vi "UHR-Fleezers Control (host) - 16.2.2v2.vi"() -> ()   [LabVIEW 2014] (continued)
        n2770 = case shown="False" w4007 {
          tunnel: [w4012 w4019] -> w4009
          tunnel: w4004 -> [w4010 w4019]
          frame False {
            n2771 = local read "Trap Pos FB Monitor\nT1 or T2"() -> (w4015:bool)
            n2772 = local read "Trap X AI1 (DMA)"() -> (w4018:T15)
            n2773 = Unbundle By Name(w4018) -> ("Set 1"=w4017:fxp<+/-,16,1>, "Set 2"=w4016:fxp<+/-,16,1>)
            n2774 = Select(t=w4017, s=w4015, f=w4016) -> (s? t:f=w4014:fxp<+/-,16,1>)
            n2775 = Not(x="Set SP Using...") -> (.not. x?=w4011:bool)
            n2776 = Select(t=w4010, s=w4011, f=w4014) -> (s? t:f=w4012:fxp<+/-,16,1>)
          }
          frame True {
          }
        }
        n2777 = xnode "Read/Write Control"("FPGA VI Reference In"=w4006, "error in"=w4005, "Trap Pos. FB SP"=w4009) -> ()  [unwired: 2 out]
        n2778 = local write "Trap Pos FB SP"(w4009) -> ()
      }
      event "Trap Pos. FB Out Scale 2^n": Value Change {
        n2779 = event-data() -> ()  [unwired: 7 out]
        n2780 = Scale By Power Of 2(n="Trap Pos. FB Out Scale 2^n", x=ext 1.0) -> (x*2^n=w4020:ext)
        n2781 = property on="Trap Pos. FB Mult Factor" class="DigNum (strict)"("Val(Sgnl)"=w4020) -> ()  [unwired: 2 in, 2 out]
      }
      event "Trap Pos FB Int Count": Value Change {
        n2782 = event-data() -> ()  [unwired: 7 out]
        n2783 = xnode "Read/Write Control"("FPGA VI Reference In"=w4023, "Trap Pos FB Int Count"="Trap Pos FB Int Count") -> ()  [unwired: 1 in, 2 out]
      }
      event "Display Saved Data": Value Change {
        n2784 = event-data() -> ()  [unwired: 7 out]
        n2785 = case shown="\"Amp Current\"" "Display Saved Data" {
          frame "Bead Seperation", Default {
            n2786 = property on="Amp current" class="WFGraph (strict)"("Visible"=FALSE) -> ()  [unwired: 2 in, 2 out]
            n2787 = property on="Trap Delta Graph" class="WFGraph (strict)"("Visible"=TRUE) -> ()  [unwired: 2 in, 2 out]
            n2788 = property on="Saved trap pos" class="WFGraph (strict)"("Visible"=FALSE) -> ()  [unwired: 2 in, 2 out]
          }
          frame "Amp Current" {
            n2789 = property on="Saved trap pos" class="WFGraph (strict)"("Visible"=FALSE) -> ()  [unwired: 2 in, 2 out]
            n2790 = property on="Trap Delta Graph" class="WFGraph (strict)"("Visible"=FALSE) -> ()  [unwired: 2 in, 2 out]
            n2791 = property on="Amp current" class="WFGraph (strict)"("Visible"=TRUE) -> ()  [unwired: 2 in, 2 out]
          }
          frame "Trap Position" {
            n2792 = property on="Saved trap pos" class="WFGraph (strict)"("Visible"=TRUE) -> ()  [unwired: 2 in, 2 out]
            n2793 = property on="Trap Delta Graph" class="WFGraph (strict)"("Visible"=FALSE) -> ()  [unwired: 2 in, 2 out]
            n2794 = property on="Amp current" class="WFGraph (strict)"("Visible"=FALSE) -> ()  [unwired: 2 in, 2 out]
          }
        }
      }
      event "Calibration": Value Change {
        n2795 = event-data() -> ()  [unwired: 7 out]
        n2796 = local read "X or Y?"() -> (w4051:bool)
        n2797 = local read "Calibration"() -> (w4048:u16)
        n2798 = Select(t="X" ("Label.Text"), s=w4051, f="Y" ("Label.Text")) -> (s? t:f=w4045:string)
        n2799 = case shown="0, Default" w4048 {
          tunnel: ["Position (V)" ("Label.Text") "Position (nm)" ("Label.Text") "Force (pN)" ("Label.Text")] -> w4042
          tunnel: [" (V)" ("Label.Text") " (nm)" ("Label.Text") " (pN)" ("Label.Text")] -> w4039
          frame 0, Default {
          }
          frame 1 {
          }
          frame 2 {
          }
        }
        n2800 = Concatenate Strings("T1 " ("Label.Text"), w4045) -> (w4041:string)
        n2801 = Concatenate Strings("T2 " ("Label.Text"), w4045) -> (w4040:string)
        n2802 = property on="Force" class="WFChart (strict)"("YScale.NameLbl.Text"=w4042) -> ()  [unwired: 2 in, 2 out]
        n2803 = Concatenate Strings("Mean" ("Label.Text"), w4039) -> (w4038:string)
        n2804 = Concatenate Strings(w4041, w4039) -> (w4037:string)
        n2805 = Concatenate Strings(w4040, w4039) -> (w4036:string)
        n2806 = Concatenate Strings("Difference" ("Label.Text"), w4039) -> (w4035:string)
        n2807 = property on="Mean" class="DigNum (strict)"("Caption.Text"=w4038) -> ()  [unwired: 2 in, 2 out]
        n2808 = property on="T1 X" class="DigNum (strict)"("Caption.Text"=w4037) -> ()  [unwired: 2 in, 2 out]
        n2809 = property on="T2 X" class="DigNum (strict)"("Caption.Text"=w4036) -> ()  [unwired: 2 in, 2 out]
        n2810 = property on="Difference" class="DigNum (strict)"("Caption.Text"=w4035) -> ()  [unwired: 2 in, 2 out]
      }
      event "Base N trap periods", "Period scale factor", "Trap osc amp (MHz)", "Cal sets to save", "# Samples/trap", "Total Counts (ticks)": Value Change {
        w4063 = u32 0 ("y")
        # "scales 0 to 2pi"
        # "Create vector of trap offset (oscillation) values."
        # "Compute oscillation period as a multiple of the trap period. Should also fit nicely as a factor of the DMA period.\nCompare ticks for accurate commensurability check."
        # "Oscillation frequency needs to be commensurate\nwith the data save time."
        # "Be commensurate with total save time/100 (or so). That way you are guaranteed you can average spectra at least 100x."
        n2811 = event-data() -> ()  [unwired: 7 out]
        n2812 = local read "Total Counts (ticks)"() -> (w4082:u16)
        n2813 = To Unsigned Long Integer(number=w4082) -> (unsigned 32bit integer=w4092:u32)
        n2814 = Multiply "Base osc period (ticks)"(x=w4092, y="Base N trap periods") -> (x*y=w4083:u32)
        n2815 = local read "# Samples/trap"() -> (w4087:u32)
        n2816 = Multiply "Scaled osc period (ticks)"(x=w4083, y="Period scale factor") -> (x*y=w4084:dbl)
        n2817 = Multiply(x="Base N trap periods", y="Period scale factor") -> (x*y=w4075:dbl)
        n2818 = local read "Cal sets to save"() -> (w4088:u32)
        n2819 = To Unsigned Quad Integer(1:w4084) -> (0:w4072:u64)
        n2820 = for "vector 0 to N -1" {
          N: w4075 -> [_]
          tunnel: [w4110] -> w4080 mode=indexing
          i -> [w4110]
        }
        n2821 = Multiply "Ticks/DMA"(x=w4087, y=w4092) -> (x*y=w4091:u32)
        n2822 = Multiply "Scaled osc period (s)"(x=w4072, y=2.5e-08) -> (x*y=w4086:dbl)
        "Trap OSC Period (s)" <- w4086
        n2823 = Reciprocal(x=w4086) -> (1/x=→"A cal freq (Hz)":dbl)
        n2824 = Multiply(x=w4080, y=6.283185307179586) -> (x*y=w4095:dbl[])
        n2825 = Quotient & Remainder(x=w4091, y=w4072) -> (x-y*floor(x/y)=w4064:u64, floor(x/y)=→"N osc / DMA":u64)
        "DMA remainder" <- w4064
        n2826 = Multiply "Total trap ticks"(x=w4088, y=w4091) -> (x*y=w4073:u32)
        n2827 = Divide(x=w4095, y=w4075) -> (x/y=w4096:dbl[])
        n2828 = Sine(x=w4096) -> (sin(x)=w4097:dbl[])
        n2829 = Quotient & Remainder(x=w4073, y=100) -> (x-y*floor(x/y)=w4067:u32, floor(x/y)=w4090:u32)
        "Total save/100 remainder" <- w4067
        n2830 = Multiply "Single period osc vector"(x=w4097, y="Trap osc amp (MHz)") -> (x*y=w4070:dbl[])
        n2831 = Quotient & Remainder(x=w4090, y=w4072) -> (x-y*floor(x/y)=w4066:u64, floor(x/y)=→"N osc/ (total save/100)":u64)
        "(total save/100) /osc period remainder" <- w4066
        n2832 = Quotient & Remainder(x=w4073, y=w4072) -> (x-y*floor(x/y)=w4065:u64, floor(x/y)=w4071:u64)
        "N trap osc periods per save" <- w4071
        "N trap osc periods per save remainder" <- w4065
        n2833 = call "IR AOM freq to word - vec.vi"("Frequency In (double vec, MHz)"=w4070) -> ("Frequency Word Out"=w4069:dbl[])
        n2834 = xnode "Read/Write Control"("FPGA VI Reference In"=w4079, "Trap osc period (pts)"=w4075, "N trap osc periods"=w4071) -> ("FPGA VI Reference Out"=w4078:T25)  [unwired: 1 in, 1 out]
        n2835 = To Quad Integer(1:w4069) -> (0:w4068:i64[])
        n2836 = Equal?(x=w4066, y=w4063) -> (x = y?=w4061:bool)
        n2837 = Equal?(x=w4067, y=w4063) -> (x = y?=w4062:bool)
        n2838 = Equal?(x=w4064, y=w4063) -> (x = y?=w4059:bool)
        n2839 = Equal?(x=w4065, y=w4063) -> (x = y?=w4060:bool)
        n2840 = flat-sequence {
          tunnel: w4068 -> [w4101]
          tunnel: w4078 -> [w4100]
          frame #0 {
            n2841 = for "Write data to fpga memory" {
              tunnel: w4100 -> [w4106]
              tunnel: w4101 -> [w4104] mode=indexing
              i -> [w4105]
              n2842 = xnode "Read/Write Control"("FPGA VI Reference In"=w4106, "Address 2"=w4105, "Data"=w4104, "Ready Write"=TRUE) -> ("FPGA VI Reference Out"=w4102:T25)  [unwired: 1 in, 1 out]
              n2843 = while {
                tunnel: w4102 -> [w4108]
                stop <- w4107 continue-if-true
                n2844 = xnode "Read/Write Control"("FPGA VI Reference In"=w4108) -> ("Ready Write"=w4107:bool)  [unwired: 1 in, 2 out]
              }
            }
            "Writing waveform to fpga memory" <- TRUE ("Writing waveform to fpga memory")
          }
          frame #1 {
            n2845 = local write "Writing waveform to fpga memory"(FALSE ("Writing waveform to fpga memory")) -> ()
          }
        }
        n2846 = Compound Arithmetic op=AND(w4062, w4061, w4060, w4059) -> (→"Good freq?":bool)
      }
      event "Osc trap cont.", "Osc traps", "T1 Osc Enable", "T2 Osc Enable": Value Change {
        n2847 = event-data() -> ()  [unwired: 7 out]
        n2848 = xnode "Read/Write Control"("FPGA VI Reference In"=w4115, "Osc trap cont."="Osc trap cont.", "Osc traps"="Osc traps", "Trap 1 osc enable"="T1 Osc Enable", "Trap 2 osc enable"="T2 Osc Enable") -> ()  [unwired: 1 in, 2 out]
      }
      event "Pressure Pump Voltage (+/-10V)": Value Change {
        n2849 = event-data() -> ()  [unwired: 7 out]
        n2850 = disable-structure shown="Disabled" {
          disable-tunnel: w4116 -> [w4117 _]
          frame Disabled {
            n2851 = disable-structure shown="Enabled" {
              disable-tunnel: w4117 -> [w4120 _]
              frame Enabled {
                n2852 = Divide(x="Pressure Pump Voltage (+/-10V)", y=10.0) -> (x/y=w4118:dbl)
                n2853 = Multiply(x=w4118, y=32767.0) -> ()  [unwired: 1 out]
                n2854 = xnode "Read/Write Control"("FPGA VI Reference In"=w4120) -> ()  [unwired: 2 in, 2 out]
              }
              frame Disabled {
              }
            }
          }
          frame Enabled {
          }
        }
      }
    }
    "error out 2" <- w2711
    n2855 = node-c288() -> ()  [unwired: 2 out]
  }
  n2856 = disable-structure shown="Disabled" {
    frame Disabled {
      n2857 = while "Duncan's play event loop" {
        stop <- w4125 stop-if-true
        n2858 = Create User Event(user event datatype=TRUE ("Boolean")) -> (user event=w4126:refnum<user-event>)  [unwired: 1 in, 1 out]
        n2859 = Create User Event(user event datatype=TRUE ("Boolean")) -> (user event=w4132:refnum<user-event>)  [unwired: 1 in, 1 out]
        n2860 = global write "Global for fluorescence simulation mean (30 samples), (power series).vi" "Red Signal"(w4126) -> ()
        n2861 = global write "Global for fluorescence simulation mean (30 samples), (power series).vi" "Green Signal"(w4132) -> ()
        n2862 = register-events(w4132, w4126) -> (reference out=w4131:refnum<event-registration>)  [unwired: 2 in, 1 out]
        n2863 = event shown="[1] \"Start assembly line\": Value Change" {
          selector: w4131 -> [_ _ _ _]
          dyn-events: _ -> [_ _ _ _]
          timeout: 100 -> [_ _ _ _]
          event Timeout {
            n2864 = event-data() -> ()  [unwired: 1 in, 2 out]
          }
          event "Start assembly line": Value Change {
            n2865 = event-data() -> ("OldVal"=w4134:bool)  [unwired: 1 in, 4 out]
            n2866 = case shown="True" w4134 {
              selector: w4134 -> [_ w4135]
              frame False {
              }
              frame True {
                n2867 = property on="Move to Position 3" class="Bool"("Val(Sgnl)"=w4135) -> ()  [unwired: 2 in, 2 out]
                n2868 = case shown="1" "Numeric" {
                  frame 0, Default {
                  }
                  frame 1 {
                    n2869 = property on="Green Laser ON" class="Bool (strict)"("Val(Sgnl)"=TRUE ("Value (Signaling)")) -> ()  [unwired: 2 in, 2 out]
                  }
                  frame 2 {
                    n2870 = property on="Red Laser ON" class="Bool (strict)"("Val(Sgnl)"=TRUE) -> ()  [unwired: 2 in, 2 out]
                  }
                }
              }
            }
          }
          event User Event {
            n2871 = event-data() -> ("Boolean"=w4139:bool)  [unwired: 1 in, 3 out]
            "Green Fluorophore" <- w4139
            n2872 = property on="Start assembly line" class="Bool"("Val(Sgnl)"=w4139) -> ()  [unwired: 2 in, 2 out]
          }
          event User Event {
            n2873 = event-data() -> ("Boolean"=w4140:bool)  [unwired: 1 in, 3 out]
            "Red Fluorophore" <- w4140
            n2874 = property on="Start assembly line" class="Bool"("Val(Sgnl)"=w4140) -> ()  [unwired: 2 in, 2 out]
          }
        }
        n2875 = property on="Get Fluorophore" class="Bool (strict)"("Val(Sgnl)"="Get Fluorophore") -> ()  [unwired: 2 in, 2 out]
        n2876 = Wait (ms)(milliseconds to wait=u32 100) -> ()  [unwired: 1 out]
        n2877 = local read "Stop All"() -> (w4124:bool)
        n2878 = Or(x=w4124, y="stop") -> (x .or. y?=w4125:bool)
      }
    }
    frame Enabled {
    }
  }
  n2879 = flat-sequence "Video" {
    tunnel: [w4151] -> w75
    tunnel: w75 -> [w4192]
    frame #0 {
      w4141 = FALSE ("File open?")
      n2880 = while {
        stop <- w4143 continue-if-true
        n2881 = call "Close Video Capture.vi"() -> ("error code OUT"=w4145:i32)
        n2882 = Equal?(x=w4145, y=0) -> (x = y?=w4143:bool)
      }
      n2883 = local write "New Video File"(w4141) -> ()
      n2884 = local write "File open?"(w4141) -> ()
      n2885 = local write "Save Video"(w4141) -> ()
      n2886 = local write "Stop All"(FALSE ("Stop All")) -> ()
    }
    frame #1 {
      n2887 = call "DMR_Init.vi"() -> ()  [unwired: 3 out]
    }
    frame #2 {
      w4146 = "DE245428202"  # MSU fleezers card #
      (unwired) "DE019116701"  # Illinois fleezers card #
      # "Setting the destination format to Mono8 makes sure that the image can be displayed in the intensity plot."
      n2888 = call "DMR_GetDevice.vi"("search string IN"=w4146) -> ("device handle OUT"=w4169:i32)  [unwired: 4 in, 2 out]
      n2889 = call "DMR_OpenDevice.vi"("device handle IN"=w4169) -> ("driver handle OUT"=w4152:i32)  [unwired: 4 out]
      n2890 = call "DMR_FindList.vi"("flags IN"=u32 0 ("flags"), "list name IN"="" ("String"), "list type IN"=T41."camera descriptions", "driver handle IN"=w4152) -> ("list handle OUT"=w4155:i32)  [unwired: 2 out]
      n2891 = call "DMR_FindList.vi"("flags IN"=u32 0 ("flags"), "list name IN"="Base", "list type IN"=T41."setting", "driver handle IN"=w4152) -> ("list handle OUT"=w4153:i32)  [unwired: 2 out]
      n2892 = call "OBJ_GetHandle.vi"("object name IN"="VideoStandard", "list handle IN"=w4155) -> ("object handle OUT"=w4149:i32)  [unwired: 3 out]
      n2893 = call "OBJ_GetHandle.vi"("object name IN"="PixelFormat", "list handle IN"=w4153) -> ("object handle OUT"=w4163:i32)  [unwired: 3 out]
      n2894 = call "OBJ_SetS.vi"("value index IN"=0, "value IN"="NTSC M", "object handle IN"=w4149) -> ()  [unwired: 2 out]
      n2895 = call "OBJ_SetS.vi"("value index IN"=0, "value IN"="Mono8" ("value"), "object handle IN"=w4163) -> ()  [unwired: 2 out]
      n2896 = call "OBJ_GetHandle.vi"("object name IN"="VideoChannel", "list handle IN"=w4153) -> ("object handle OUT"=w4159:i32)  [unwired: 3 out]
      n2897 = while {
        tunnel: [w4173] -> w4151
        tunnel: w4152 -> [w4170]
        stop <- w4171 continue-if-true
        n2898 = call "DMR_ImageRequestSingle.vi"("request control IN"=0, "driver handle IN"=w4170) -> ("error code OUT"=w4172:i32, "driver handle OUT"=w4173:i32)  [unwired: 2 out]
        n2899 = Equal To 0?(x=w4172) -> (x = 0?=w4171:bool)
      }
      n2900 = call "OBJ_SetI.vi"("value index IN"=0, "value IN"="Video channel", "object handle IN"=w4159) -> ()  [unwired: 2 out]
    }
    frame #3 {
      w4180 = T22 0 items=["Grayscale (U8)", "Grayscale (I16)", "Grayscale (SGL)", "Complex (CSG)", "RGB (U32)", "HSL (U32)", "RGB (U64)"] ("Image Type")
      w4188 = T22 0 items=["Grayscale (U8)", "Grayscale (I16)", "Grayscale (SGL)", "Complex (CSG)", "RGB (U32)", "HSL (U32)", "RGB (U64)"] ("Image Type")
      n2901 = call "IMAQ AVI2 Get Codec Names"() -> ("Codec Names"=w4175:string[])  [unwired: 10 in, 1 out]
      "Installed Codec Names" <- w4175
      n2902 = for "Create Greyscale map" {
        N: 256 -> [_]
        tunnel: [w4194] -> w4177 mode=indexing
        workers-P: _ -> [_]
        i -> [w4197]
        n2903 = To Unsigned Byte Integer(number=w4197) -> (unsigned 8bit integer=w4193:u8)
        n2904 = Join Numbers(hi=w4193, lo=w4193) -> ((hi.lo)=w4196:u16)
        n2905 = Join Numbers(hi=w4193, lo=w4193) -> ((hi.lo)=w4195:u16)
        n2906 = Join Numbers(hi=w4196, lo=w4195) -> ((hi.lo)=w4194:u32)
      }
      n2907 = property on="Codec choice" class="CmbBox"("Strings[]"=w4175) -> ()  [unwired: 2 in, 2 out]
      n2908 = call "IMAQ Create"("Image Name"="Scaled video", "Image Type"=w4180) -> ("New Image"=w4179:T2)  [unwired: 2 in, 2 out]
      n2909 = call "IMAQ Create"("Image Name"="Main video", "Image Type"=w4188) -> ("New Image"=w4189:T2)  [unwired: 2 in, 2 out]
      n2910 = node-c288(0 ("Processor")) -> (w4187:T28)  [unwired: 3 out]
      n2911 = Initialize Array(u32 0 ("Window Number (0...15)"), 480 ("dimension size"), 640 ("dimension size")) -> (w4182:u32[][])
      n2912 = timed-loop {
        tunnel: w4192 -> [w4214]
        tunnel: [w4213] -> w4191
        tunnel: w4189 -> [w4212]
        timing: w4187 -> [_]
        timing-out: [_] -> w4186
        tunnel: w4182 -> [w4205]
        tunnel: w4179 -> [w4203]
        tunnel: w4177 -> [w4202]
        stop <- w4204 stop-if-true
        # "This block performs the \nactual image capture."
        n2913 = node-c288() -> (→"Finished Late? [i-1]":bool)  [unwired: 5 out]
        n2914 = local read "Stop All"() -> (w4204:bool)
        n2915 = feedback #2(T42 refnum ("AVI Refnum")) -> (w4210:T42)
        n2916 = case shown="True" "New Video File" {
          tunnel: [w4227 w4228] -> w4201
          tunnel: w4210 -> [w4227 w4229]
          frame False {
          }
          frame True {
            n2917 = flat-sequence {
              tunnel: w4229 -> [w4231]
              tunnel: [w4233] -> w4228
              frame #0 {
                n2918 = local read "File open?"() -> (w4230:bool)
                n2919 = case shown="True" w4230 {
                  tunnel: w4231 -> [_ w4232]
                  frame False {
                  }
                  frame True {
                    n2920 = call "IMAQ AVI2 Close"("AVI Refnum"=w4232) -> ()  [unwired: 10 in, 1 out]
                  }
                }
              }
              frame #1 {
                n2921 = local write "New Video File"(FALSE ("New Video File")) -> ()
                n2922 = call "Create new save file.vi"("Ext"=".avi" ("string"), "Index In"="Video Index") -> ("Path Out"=w4236:path, "Index Out"=w4238:dbl)  [unwired: 1 in]
                "Path Out" <- w4236
                n2923 = local write "Video Index"(w4238) -> ()
                n2924 = call "IMAQ AVI2 Create"("Codec"="Codec choice", "Frames Per Second"=u32 30, "AVI Path"=w4236) -> ("AVI Refnum"=w4233:T42)  [unwired: 7 in, 1 out]
                "File open?" <- TRUE ("Files open?")
              }
            }
          }
        }
        n2925 = feedback-in #2(w4201) -> ()
        n2926 = call "DMR_ImageRequestWaitFor.vi"("queue number IN"=0, "timeout(ms) IN"=500, "driver handle IN"=w4214) -> ("error code OUT"=w4218:i32, "request number OUT"=w4215:i32, "driver handle OUT"=w4216:i32)
        n2927 = Equal To 0?(x=w4218) -> (x = 0?=w4217:bool)
        n2928 = Reciprocal(x="Video Capture Rate (Hz)") -> (1/x=w4208:dbl)
        n2929 = Multiply(x=w4208, y=1000.0) -> (x*y=w4206:dbl)
        n2930 = case shown="True" w4217 {
          tunnel: w4216 -> [w4242 w4279]
          tunnel: w4215 -> [_ w4278]
          tunnel: [w4242 w4275] -> w4213
          tunnel: w4212 -> [_ w4261]
          tunnel: w4205 -> [_ w4264]
          tunnel: w4201 -> [_ w4244]
          tunnel: w4203 -> [_ w4258]
          tunnel: w4202 -> [_ w4257]
          frame False {
          }
          frame True {
            w4269 = u32 0 ("X-offset IN")
            n2931 = call "DMR_GetImageRequestBufferData.vi"("driver handle IN"=w4279, "request number IN"=w4278) -> ("width OUT"=w4268:i32, "height OUT"=w4267:i32, "driver handle OUT"=w4274:i32, "request number OUT"=w4273:i32, "bytes per pixel OUT"=w4270:i32)  [unwired: 13 out]
            n2932 = call "DMR_GetImageRequestBufferImageData.vi"("driver handle IN"=w4274, "request number IN"=w4273, "bytes per pixel IN"=w4270, "X-offset IN"=w4269, "Y-offset IN"=w4269, "height IN"=w4267, "width IN"=w4268) -> ("driver handle OUT"=w4272:u32, "request number OUT"=w4271:u32, "image OUT"=w4250:u32[][])  [unwired: 10 out]
            n2933 = Transpose 2D Array(2D array=w4250) -> (transposed array=w4256:u32[][])
            n2934 = Select(t=w4256, s="Flip Y (or X)", f=w4250) -> (s? t:f=w4255:u32[][])
            n2935 = call "DMR_ImageRequestUnlock.vi"("request number IN"=w4271, "driver handle IN"=w4272) -> ("driver handle OUT"=w4277:i32)  [unwired: 1 in, 2 out]
            n2936 = for {
              tunnel: w4255 -> [w4314] mode=indexing
              tunnel: [w4313] -> w4253 mode=indexing
              n2937 = Reverse 1D Array(array=w4314) -> (reversed array=w4313:u32[])
            }
            n2938 = call "DMR_ImageRequestSingle.vi"("request control IN"=0, "driver handle IN"=w4277) -> ("driver handle OUT"=w4275:i32)  [unwired: 3 out]
            n2939 = Transpose 2D Array(2D array=w4253) -> (transposed array=w4254:u32[][])
            n2940 = Select(t=w4254, s="Flip Y (or X)", f=w4253) -> (s? t:f=w4251:u32[][])
            n2941 = Select(t=w4251, s="Flip Image", f=w4250) -> (s? t:f=w4248:u32[][])
            n2942 = case shown="True" "Averaging" {
              tunnel: w4248 -> [w4325 w4330]
              tunnel: [w4325 w4329] -> w4262
              tunnel: w4264 -> [_ w4327]
              frame False {
              }
              frame True {
                (unwired) 1
                w4335 = 1
                n2943 = feedback #3(w4327) -> (w4326:u32[][])
                n2944 = Add(x=w4330, y=w4326) -> (x+y=w4331:u32[][])
                n2945 = Select(t=w4327, s="Reset Averaging", f=w4331) -> (s? t:f=w4333:u32[][])
                n2946 = feedback-in #3(w4333) -> ()
                n2947 = feedback #4(w4335) -> (w4328:i32)
                n2948 = Divide(x=w4331, y=w4328) -> (x/y=w4332:dbl[][])
                n2949 = Increment(x=w4328) -> (x+1=w4336:i32)
                n2950 = To Unsigned Long Integer(number=w4332) -> (unsigned 32bit integer=w4329:u32[][])
                n2951 = Select(t=w4335, s="Reset Averaging", f=w4336) -> (s? t:f=w4334:i32)
                n2952 = feedback-in #4(w4334) -> ()
              }
            }
            n2953 = case shown="True" "Zoom video window" {
              tunnel: w4262 -> [_ w4293]
              tunnel: w4258 -> [_ w4292]
              frame False {
              }
              frame True {
                n2954 = To Double Precision Float(number=w4293) -> (double precision float=w4290:dbl[][])
                n2955 = In Range and Coerce(upper limit="Intensity Upper", x=w4290, lower limit="Intensity Lower") -> (coerced(x)=w4289:dbl[][])  [unwired: 1 out]
                n2956 = Subtract(x="Intensity Upper", y="Intensity Lower") -> (x-y=w4286:dbl)
                n2957 = Subtract(x=w4289, y="Intensity Lower") -> (x-y=w4287:dbl[][])
                n2958 = Divide(x=w4287, y=w4286) -> (x/y=w4288:dbl[][])
                n2959 = Multiply(x=255.0, y=w4288) -> (x*y=w4284:dbl[][])
                n2960 = To Unsigned Byte Integer(number=w4284) -> (unsigned 8bit integer=w4291:u8[][])
                n2961 = call "IMAQ ArrayToImage"("Image Pixels (U8)"=w4291, "Image"=w4292) -> ("Image Out"=w4280:T2)  [unwired: 4 in, 5 out]
                n2962 = First Call?() -> (First Call?: T/F=w4281:bool)
                n2963 = case shown="True" w4281 {
                  tunnel: w4280 -> [w4294 w4305]
                  frame False {
                    n2964 = flat-sequence {
                      tunnel: w4294 -> [w4300]
                      frame #0 {
                        w4297 = FALSE ("Get/Set Status? (Set)")
                        w4296 = 0 ("Window Number (0...15)")
                        n2965 = call "IMAQ WindSize"("Get/Set Status? (Set)"=w4297, "Window Number"=w4296) -> ("Width & Height out"=→"Window Size":cluster{"Width":i32, "Height":i32})  [unwired: 4 in, 2 out]
                        n2966 = call "IMAQ WindMove"("Window Number (0...15)"=w4296, "Get/Set Status? (Set)"=w4297) -> ("Coordinates (screen)"=→"Window Position":cluster{"X Position":i32, "Y Position":i32})  [unwired: 3 in, 1 out]
                        n2967 = call "IMAQ WindDraw"("Resize to Image Size? (Y)"=FALSE, "Window Number (0...15)"=w4296, "Image"=w4300) -> ()  [unwired: 7 in, 2 out]
                      }
                      frame #1 {
                        n2968 = call "IMAQ WindZoom 2"("Center Point"="Center Point", "Zoom to Fit? (False)"=FALSE, "Zoom Factor"="Zoom Factor") -> ()  [unwired: 5 in, 4 out]
                      }
                    }
                  }
                  frame True {
                    n2969 = flat-sequence {
                      tunnel: w4305 -> [w4308]
                      tunnel: [w4306] -> w4304
                      tunnel: w4304 -> [w4310]
                      frame #0 {
                        w4307 = TRUE ("Resize to Image Size? (Y)")
                        w4306 = 0 ("Window Number (0...15)")
                        n2970 = call "IMAQ WindNonTearing"("Window Number"=w4306, "NonTearing? (True)"=w4307) -> ()  [unwired: 8 in, 2 out]
                        n2971 = call "IMAQ WindDraw"("Resize to Image Size? (Y)"=w4307, "Window Number (0...15)"=w4306, "Image"=w4308) -> ()  [unwired: 7 in, 2 out]
                      }
                      frame #1 {
                        n2972 = call "IMAQ WindSize"("Scrollbars? (N)"=FALSE, "Width & Height"="Initial Window Size", "Window Number"=w4310) -> ()  [unwired: 3 in, 3 out]
                        n2973 = call "IMAQ WindMove"("Window Number (0...15)"=w4310, "Coordinates (screen)"="Initial Window Position") -> ()  [unwired: 3 in, 2 out]
                      }
                    }
                  }
                }
              }
            }
            n2974 = To Unsigned Byte Integer(number=w4262) -> (unsigned 8bit integer=w4260:u8[][])
            n2975 = call "IMAQ ArrayToImage"("Image Pixels (U8)"=w4260, "Image"=w4261) -> ("Image Out"=w4259:T2)  [unwired: 4 in, 5 out]
            "Primary Video Display" <- w4259
            n2976 = Not(x="Close Video File") -> (.not. x?=w4246:bool)
            n2977 = And(x="Save Video", y=w4246) -> (x .and. y?=w4243:bool)
            n2978 = case shown="True" "Save Image" {
              tunnel: w4260 -> [_ w4339]
              tunnel: w4257 -> [_ w4338]
              frame False {
              }
              frame True {
                n2979 = call <vilib>:"Flatten Pixmap.vi"("colors"=w4338, "8-bit pixmap"=w4339) -> ("image data"=w4345:T43)  [unwired: 4 in, 5 out]
                n2980 = call "Create new save file.vi"("Insert"="video_frame_" ("string"), "Ext"=".bmp" ("string"), "Index In"="Image Index") -> ("Path Out"=w4341:path, "Index Out"=w4346:dbl)
                n2981 = Increment(x=w4346) -> (x+1=w4340:dbl)
                n2982 = local write "Image Index"(w4340) -> ()
                n2983 = call <vilib>:"Write BMP File.vi"("image data"=w4345, "path to BMP file"=w4341) -> ()  [unwired: 1 in, 9 out]
              }
            }
            n2984 = case shown="True" w4243 {
              tunnel: w4244 -> [w4316 w4321]
              tunnel: w4259 -> [_ w4320]
              tunnel: "Close Video File" -> [w4315 _]
              frame False {
                n2985 = case shown="True" w4315 {
                  tunnel: w4316 -> [_ w4317]
                  frame False {
                  }
                  frame True {
                    w4318 = FALSE ("Save Video")
                    n2986 = call "IMAQ AVI2 Close"("AVI Refnum"=w4317) -> ()  [unwired: 10 in, 1 out]
                    n2987 = local write "File open?"(w4318) -> ()
                    n2988 = local write "Save Video"(w4318) -> ()
                  }
                }
              }
              frame True {
                n2989 = local read "File open?"() -> (w4319:bool)
                n2990 = case shown="True" w4319 {
                  tunnel: w4321 -> [_ w4324]
                  tunnel: w4320 -> [_ w4323]
                  frame False {
                    n2991 = local write "New Video File"(TRUE ("New Video File")) -> ()
                  }
                  frame True {
                    n2992 = call "IMAQ AVI2 Write Frame"("Image"=w4323, "AVI Refnum"=w4324) -> ()  [unwired: 7 in, 3 out]
                  }
                }
              }
            }
          }
        }
        n2993 = node-c288(w4206, "Deadline (ms)") -> ()  [unwired: 1 out]
      }
      n2994 = node-c288(w4186) -> ()  [unwired: 1 out]
      n2995 = call "DMR_CloseDevice.vi"("driver handle IN"=w4191) -> ()  [unwired: 1 in, 4 out]
    }
    frame #4 {
      n2996 = call "DMR_Close.vi"() -> ()  [unwired: 1 out]
    }
  }
  n2997 = node-c288(w45) -> ()  [unwired: 1 out]
  n2998 = node-c288(w84) -> ()  [unwired: 1 out]
  n2999 = node-c288(w86) -> ()  [unwired: 1 out]
  n3000 = node-c288(w73) -> ()  [unwired: 1 out]
  n3001 = disable-structure shown="Disabled" {
    disable-tunnel: w77 -> [w4352 _]
    disable-tunnel: w76 -> [w4351 _]
    frame Disabled {
      n3002 = VISA Close(VISA resource name=w4352, error in (no error)=w4351) -> (error out=w4353:errorcluster)
      n3003 = call <vilib>:"Simple Error Handler.vi"("error in (no error)"=w4353) -> ()  [unwired: 1 in, 8 out]
    }
    frame Enabled {
    }
  }
  n3004 = property on="Saved trap pos" class="WFGraph (strict)"("Visible"=FALSE) -> ()  [unwired: 2 in, 2 out]
  n3005 = property on="Trap Delta Graph" class="WFGraph (strict)"("Visible"=TRUE) -> ()  [unwired: 2 in, 2 out]
  n3006 = node-c288(w82) -> ()  [unwired: 1 out]
  n3007 = Unbundle By Name("sound format") -> ("sample rate (S/s)"=w23:dbl)
  n3008 = call <vilib>:"Sound Output Configure.vi"("number of samples/ch"="number of samples/ch", "sample mode"="sample mode", "sound format"="sound format", "device ID"="device ID") -> ("task ID"=w27:T44)  [unwired: 6 in, 1 out]
  n3009 = local read "DMA Update Period (s)"() -> (w24:dbl)
  n3010 = Multiply(x=w24, y=w23) -> (x*y=w22:dbl)
  n3011 = for "Sound time base" {
    N: w22 -> [_]
    tunnel: [w4354] -> w25 mode=indexing
    i -> [w4354]
  }
  n3012 = Reciprocal(x=w23) -> (1/x=w21:dbl)
  n3013 = Multiply(x=w25, y=w21) -> (x*y=w20:dbl[])
  n3014 = timed-loop "Main data acquisition loop (get data, process data for display, and save data to disk)" {
    tunnel: w16 -> [w4697]
    tunnel: w40 -> [w4696]
    tunnel: [w4725] -> w98
    tunnel: [w4720] -> w97
    timing: w91 -> [_]
    timing-out: [_] -> w90
    tunnel: w67 -> [w4585]
    tunnel: [w4423] -> w31
    tunnel: w27 -> [w4422]
    tunnel: w23 -> [w4420]
    tunnel: w22 -> [w4419]
    tunnel: w21 -> [w4418]
    tunnel: w20 -> [w4417]
    stop <- "Stop All" stop-if-true
    w4505 = "Initialize"
    # "Fluorescence lifetime measurement"
    # "List of channels in order (X or Y only):\nT1 X (mV)\nT2 X (mV)\nT1 X (nm)\nT2 X (nm)\nT1 FX (pN)\nT2 FX (pN)\nPosition Difference (nm)\nAPD1\nAPD2\nAPD3"
    # "T2 sum"
    # "T1 sum"
    # "Fluorescence data into FIFO for external control vi's\n(e.g., fluorescence triggering) - Duncan Nall"
    n3015 = node-c288() -> ()  [unwired: 2 out]
    n3016 = First Call?() -> (First Call?: T/F=w4540:bool)
    n3017 = Or(x="Reset", y=w4540) -> (x .or. y?=w4541:bool)
    n3018 = local read "Flushing P1"() -> (w4463:bool)
    n3019 = case "Reset data stream (manual reset or at begining of some rastering and imaging)" shown="True" w4541 {
      tunnel: w4697 -> [w5835 w5844]
      tunnel: w4696 -> [w5834 w5843]
      tunnel: [w5835 w5838] -> w4396
      tunnel: [w5834 w5837] -> w4397
      frame False {
      }
      frame True {
        w5841 = TRUE ("AI to FIFO")
        n3020 = local write "Overflow (data lost)"(FALSE ("Overflow (data lost)")) -> ()
        n3021 = local write "Reset"(FALSE ("Reset")) -> ()
        n3022 = call "reset FPGA DMA.vi"("error in"=w5843, "FPGA VI Reference In"=w5844) -> ("error out"=w5839:errorcluster, "FPGA VI Reference Out"=w5840:T25)
        n3023 = xnode "Read/Write Control"("FPGA VI Reference In"=w5840, "error in"=w5839, "AI to FIFO"=w5841, "APD to FIFO"=w5841) -> ("FPGA VI Reference Out"=w5838:T25, "error out"=w5837:errorcluster)
      }
    }
    n3024 = case shown="True" w4463 {
      frame False {
      }
      frame True {
        n3025 = local read "Flush rate (uL/m) P1"() -> (w4870:dbl)
        n3026 = local read "HP1 Flush Time (s)"() -> (w4879:dbl)
        n3027 = local read "DMA Update Period (s)"() -> (w4873:dbl)
        n3028 = Divide(x=w4870, y=60.0) -> (x/y=w4871:dbl)
        n3029 = Divide(x=w4879, y=w4873) -> (x/y=w4868:dbl)
        n3030 = feedback #5(0) -> (w4877:i32)
        n3031 = Increment(x=w4877) -> (x+1=w4867:i32)
        n3032 = Greater?(x=w4867, y=w4868) -> (0:w4876:bool)
        n3033 = Compound Arithmetic op=MULTIPLY(w4873, w4867, w4871) -> (→"P1 Flush Volume (uL)":dbl)
        n3034 = Divide(x=w4867, y=w4868) -> (x/y=→"P1 Flushing Bar":dbl)
        n3035 = case shown="True" w4876 {
          tunnel: w4867 -> [w4880 _]
          tunnel: [w4880 0] -> w4875
          frame False {
          }
          frame True {
            w4881 = FALSE ("Flushing P1")
            n3036 = local write "Inject Pump 1"(w4881) -> ()
            n3037 = local write "Flushing P1"(w4881) -> ()
            n3038 = property on="Clear Volume P1" class="Bool (strict)"("Val(Sgnl)"=TRUE ("Value (Signaling)")) -> ()  [unwired: 2 in, 2 out]
          }
        }
        n3039 = feedback-in #5(w4875) -> ()
      }
    }
    n3040 = Or(x="Start AOD Scan", y="Trap Raster Scan") -> (x .or. y?=w4659:bool)
    n3041 = case "Start active calibration (oscillate traps precisely)" shown="True" "Active Cal" {
      tunnel: w4397 -> [w4784 w4792]
      tunnel: w4396 -> [w4783 w4793]
      tunnel: [w4784 w4789] -> w4395
      tunnel: [w4783 w4790] -> w4394
      frame False {
      }
      frame True {
        w4785 = TRUE ("APD to FIFO")
        n3042 = call "reset FPGA DMA.vi"("error in"=w4792, "FPGA VI Reference In"=w4793) -> ("error out"=w4786:errorcluster, "FPGA VI Reference Out"=w4787:T25)
        n3043 = local write "Active Cal"(FALSE ("Active Cal")) -> ()
        n3044 = local write "Save Calibration"(TRUE ("Save Calibration")) -> ()
        n3045 = xnode "Read/Write Control"("FPGA VI Reference In"=w4787, "error in"=w4786, "AI to FIFO"=w4785, "APD to FIFO"=w4785, "Initiate trap osc"=w4785) -> ("FPGA VI Reference Out"=w4790:T25, "error out"=w4789:errorcluster)
      }
    }
    n3046 = case "Start AOM raster scan" shown="True" w4659 {
      tunnel: w4394 -> [w5685 w5695]
      tunnel: w4395 -> [w5684 w5694]
      tunnel: [w5685 w5688] -> w4692
      tunnel: [w5684 w5687] -> w4691
      frame False {
      }
      frame True {
        n3047 = case shown="True" "Restart DMA? (AOD)" {
          tunnel: [w5733 w5735] -> w5689
          tunnel: [w5732 w5734] -> w5690
          tunnel: w5695 -> [w5733 w5737]
          tunnel: w5694 -> [w5732 w5736]
          frame False {
          }
          frame True {
            n3048 = local write "Overflow (data lost)"(FALSE ("Overflow (data lost)")) -> ()
            n3049 = call "reset FPGA DMA.vi"("error in"=w5736, "FPGA VI Reference In"=w5737) -> ("error out"=w5734:errorcluster, "FPGA VI Reference Out"=w5735:T25)
          }
        }
        n3050 = local write "Trap Raster Scan"(FALSE ("Trap Raster Scan")) -> ()
        n3051 = case shown="True" "Move MCL Also?" {
          tunnel: w5690 -> [w5698 w5727]
          tunnel: w5689 -> [w5699 w5728]
          tunnel: [w5697 w5731] -> w5688
          tunnel: [w5696 w5730] -> w5687
          frame False {
            w5700 = TRUE ("AI to FIFO")
            n3052 = xnode "Read/Write Control"("FPGA VI Reference In"=w5699, "error in"=w5698, "AI to FIFO"=w5700, "APD to FIFO"=w5700, "Start scan"=w5700) -> ("FPGA VI Reference Out"=w5697:T25, "error out"=w5696:errorcluster)
          }
          frame True {
            w5724 = FALSE ("1D or 2D Scan?")
            w5729 = TRUE ("AI to FIFO")
            # "Count for MCL loop"
            # "N total cycles"
            # "N steps"
            # "V_int"
            n3053 = local read "Scan Range (nm)"() -> (w5706:dbl)
            n3054 = local read "Number of F/B Scans (AOD)"() -> (w5723:u16)
            n3055 = Sign(1:w5706) -> (0:w5705:dbl)
            n3056 = Compound Arithmetic op=MULTIPLY(w5706, "MCL Step Position Ratio", "MCL/AOM Scale Tweak") -> (w5710:dbl)
            n3057 = Negate(x=w5705) -> (-x=w5702:dbl)
            n3058 = Multiply(x=w5702, y="MCL Step Increment (V_int)") -> (x*y=w5704:dbl)
            n3059 = Divide(x=w5710, y="MCL X Cal (nm/V)") -> (x/y=w5716:dbl)
            n3060 = Multiply(x=32767.0 ("y"), y=w5716) -> (x*y=w5722:dbl)
            n3061 = local read "Total Counts (ticks)"() -> (w5707:u16)
            n3062 = local read "Cycles/step (AOD)"() -> (w5718:u64)
            n3063 = local read "Scan steps (AOD)"() -> (w5719:u64)
            n3064 = Divide(x=w5722, y=10.0) -> (x/y=w5715:dbl)
            n3065 = Divide(x=w5715, y="MCL Step Increment (V_int)") -> (x/y=w5713:dbl)
            n3066 = Absolute Value(x=w5713) -> (abs(x)=w5701:dbl)
            n3067 = Compound Arithmetic op=MULTIPLY(w5719, w5718, w5707) -> (w5714:u64)
            n3068 = local write "wait to reset values"(w5729) -> ()
            n3069 = local write "MCL Scanning"(w5729) -> ()
            n3070 = Divide(x=w5714, y=w5701) -> (x/y=w5711:dbl)
            "MCL Count" <- w5711
            n3071 = xnode "Read/Write Control"("FPGA VI Reference In"=w5728, "error in"=w5727, "Scan steps (MCL)"=w5701, "Number of scans (MCL)"=w5723, "Cycles per step (MCL)"=u64 1, "Scan freq.  increment (MCL)"=w5704, "1D or 2D Scan?"=w5724, "MCL Scan Axis"=w5724, "Cont. Scan (MCL)"=w5724, "MCL count"=w5711) -> ("FPGA VI Reference Out"=w5726:T25, "error out"=w5725:errorcluster)
            n3072 = xnode "Read/Write Control"("FPGA VI Reference In"=w5726, "error in"=w5725, "AI to FIFO"=w5729, "APD to FIFO"=w5729, "Start scan"=w5729, "Start scan (MCL)"=w5729) -> ("FPGA VI Reference Out"=w5731:T25, "error out"=w5730:errorcluster)
          }
        }
        "Raster Scanning..." <- TRUE ("Scanning...")
      }
    }
    n3073 = local read "Flushing P3"() -> (w4464:bool)
    n3074 = case "Keep track of when Harvard Pump 3 is done flushing" shown="True" w4464 {
      frame False {
      }
      frame True {
        n3075 = local read "Flush rate (uL/m) P3"() -> (w4887:dbl)
        n3076 = local read "DMA Update Period (s)"() -> (w4889:dbl)
        n3077 = local read "HP3 Flush Time (s)"() -> (w4896:dbl)
        n3078 = Divide(x=w4887, y=60.0) -> (x/y=w4885:dbl)
        n3079 = feedback #6(0) -> (w4894:i32)
        n3080 = Increment(x=w4894) -> (x+1=w4888:i32)
        n3081 = Divide(x=w4896, y=w4889) -> (x/y=w4890:dbl)
        n3082 = Greater?(x=w4888, y=w4890) -> (0:w4893:bool)
        n3083 = Compound Arithmetic op=MULTIPLY(w4889, w4888, w4885) -> (→"P3 Flush Volume (uL)":dbl)
        n3084 = case shown="True" w4893 {
          tunnel: w4888 -> [w4897 _]
          tunnel: [w4897 0] -> w4892
          frame False {
          }
          frame True {
            w4898 = FALSE ("Flushing P3")
            n3085 = local write "Inject Pump 3"(w4898) -> ()
            n3086 = local write "Flushing P3"(w4898) -> ()
            n3087 = property on="Clear Volume P3" class="Bool (strict)"("Val(Sgnl)"=TRUE ("Value (Signaling)")) -> ()  [unwired: 2 in, 2 out]
          }
        }
        n3088 = feedback-in #6(w4892) -> ()
        n3089 = Divide(x=w4888, y=w4890) -> (x/y=→"P3 Flushing Bar":dbl)
      }
    }
    n3090 = And(x="Save scans", y=w4659) -> (x .and. y?=w4690:bool)
    n3091 = local read "Tick value (ns)"() -> (w4377:dbl)
    n3092 = local read "Measuring lifetimes"() -> (w4378:bool)
    n3093 = local read "Blue Laser ON"() -> (w4374:bool)
    n3094 = And(x=w4378, y=w4374) -> (x .and. y?=w4375:bool)
    n3095 = Compound Arithmetic op=OR("Start MCL Scan", "Confocal Image", "Confocal Linescan") -> (w4657:bool)
    n3096 = And(x="Save Data (MCL)", y=w4657) -> (x .and. y?=w4689:bool)
    n3097 = case "Start MCL raster scan" shown="True" w4657 {
      tunnel: w4692 -> [w5297 w5313]
      tunnel: w4691 -> [w5296 w5312]
      tunnel: [w5297 w5308] -> w4384
      tunnel: [w5296 w5307] -> w4584
      tunnel: [FALSE w5306] -> w4675
      tunnel: "Start MCL Scan" -> [_ w5301]
      tunnel: "Confocal Image" -> [_ w5300]
      tunnel: "Confocal Linescan" -> [_ _]
      frame False {
      }
      frame True {
        w5306 = TRUE
        n3098 = case shown="True" "Restart DMA? (MCL)" {
          tunnel: [w5358 w5360] -> w5311
          tunnel: [w5357 w5359] -> w5310
          tunnel: w5313 -> [w5358 w5363]
          tunnel: w5312 -> [w5357 w5362]
          frame False {
          }
          frame True {
            n3099 = call "reset FPGA DMA.vi"("error in"=w5362, "FPGA VI Reference In"=w5363) -> ("error out"=w5359:errorcluster, "FPGA VI Reference Out"=w5360:T25)
            n3100 = local write "Overflow (data lost)"(FALSE ("Overflow (data lost)")) -> ()
          }
        }
        n3101 = case shown="False" w5301 {
          selector: w5301 -> [_ w5317]
          tunnel: w5300 -> [w5316 _]
          tunnel: [w5316 w5317] -> w5299
          frame False {
            n3102 = property on="2D or 1D Scan" class="Bool (strict)"("Val(Sgnl)"=w5316) -> ()  [unwired: 2 in, 2 out]
            n3103 = property on="Confocal Image" class="Bool (strict)"("Value"=FALSE ("Start Confocal Map")) -> ()  [unwired: 2 in, 2 out]
          }
          frame True {
          }
        }
        n3104 = local write "MCL Scanning"(w5306) -> ()
        n3105 = local read "AO1"() -> (w5303:dbl)
        n3106 = local read "AO2"() -> (w5302:dbl)
        n3107 = case shown="True" "Center Scan" {
          tunnel: w5311 -> [w5324 w5356]
          tunnel: w5310 -> [w5323 w5355]
          tunnel: [w5322 w5354] -> w5308
          tunnel: [w5321 w5353] -> w5307
          tunnel: [w5319 w5340] -> w5305
          tunnel: [w5318 w5339] -> w5304
          tunnel: w5303 -> [w5319 w5345]
          tunnel: w5302 -> [w5318 w5348]
          tunnel: w5299 -> [_ _]
          frame False {
            w5320 = TRUE ("AI to FIFO")
            n3108 = xnode "Read/Write Control"("FPGA VI Reference In"=w5324, "error in"=w5323, "AI to FIFO"=w5320, "APD to FIFO"=w5320, "Start scan (MCL)"=w5320) -> ("FPGA VI Reference Out"=w5322:T25, "error out"=w5321:errorcluster)
          }
          frame True {
            w5352 = TRUE ("AI to FIFO")
            n3109 = local read "Scan steps (MCL)"() -> (w5331:u64)
            n3110 = local read "Scan lines (y)"() -> (w5327:u64)
            n3111 = local read "Fast Scan Dir"() -> (w5338:bool)
            n3112 = local read "Actual MCL Inc (V)"() -> (w5328:dbl)
            n3113 = Decrement(x=w5327) -> (x-1=w5326:u64)
            n3114 = Decrement(x=w5331) -> (x-1=w5330:u64)
            n3115 = Multiply(x=w5328, y=w5326) -> (x*y=w5325:dbl)
            n3116 = Divide(x=w5325, y=2.0) -> (x/y=w5335:dbl)
            n3117 = Multiply(x=w5328, y=w5330) -> (x*y=w5329:dbl)
            n3118 = Divide(x=w5329, y=2.0) -> (x/y=w5334:dbl)
            n3119 = Select(t=w5334, s=w5338, f=w5335) -> (s? t:f=w5333:dbl)
            n3120 = Select(t=w5335, s=w5338, f=w5334) -> (s? t:f=w5337:dbl)
            n3121 = Subtract(x=w5345, y=w5337) -> (x-y=w5336:dbl)
            n3122 = Subtract(x=w5348, y=w5333) -> (x-y=w5332:dbl)
            n3123 = local read "2D or 1D Scan"() -> (w5350:bool)
            n3124 = Not(x=w5338) -> (.not. x?=w5344:bool)
            n3125 = Not(x=w5350) -> (.not. x?=w5346:bool)
            n3126 = And(x=w5338, y=w5346) -> (x .and. y?=w5347:bool)
            n3127 = And(x=w5346, y=w5344) -> (x .and. y?=w5349:bool)
            n3128 = Select(t=w5348, s=w5349, f=w5332) -> (s? t:f=w5339:dbl)
            n3129 = Select(t=w5345, s=w5347, f=w5336) -> (s? t:f=w5340:dbl)
            n3130 = call "Volt to I16.vi"("Voltage In"=w5340) -> ("I16 Voltage Out"=w5343:i16)
            n3131 = call "Volt to I16.vi"("Voltage In"=w5339) -> ("I16 Voltage Out"=w5342:i16)
            n3132 = xnode "Read/Write Control"("FPGA VI Reference In"=w5356, "error in"=w5355, "AI to FIFO"=w5352, "APD to FIFO"=w5352, "Start scan (MCL)"=w5352, "AO1"=w5343, "AO2"=w5342) -> ("FPGA VI Reference Out"=w5354:T25, "error out"=w5353:errorcluster)
          }
        }
        "Initial Y" <- w5305
        "Initial X" <- w5304
        n3133 = local write "Tab Control 6"(T49."Imaging" ("Tab Control 6")) -> ()
        "wait to reset values" <- w5306
      }
    }
    n3134 = xnode "Read/Write Control"("FPGA VI Reference In"=w4384) -> ("FPGA VI Reference Out"=w4383:T25, "lifetime (ticks)"=w4380:u16, "lifetime events in fifo"=w4382:u16, "Lifetime to FIFO"=→"Lifetime to FIFO":bool)  [unwired: 1 in, 1 out]
    "Lifetime (ticks)" <- w4380
    "Lifetime events in FIFO" <- w4382
    n3135 = Compound Arithmetic op=MULTIPLY(0.001 ("value"), w4377, w4380) -> (→"Lifetime (us)":dbl)
    n3136 = case shown="True" w4375 {
      tunnel: w4383 -> [_ w4758]
      tunnel: w4382 -> [_ w4751]
      frame False {
      }
      frame True {
        # "make sure no zeros"
        n3137 = xnode "Invoke Method"("FPGA VI Reference In"=w4758, "Number of Elements"=w4751, "Timeout (ms)"=-1) -> ("FPGA VI Reference Out"=w4754:T25, "Data"=w4755:u16[])  [unwired: 1 in, 2 out]
        n3138 = local read "Tick value (ns)"() -> (w4747:dbl)
        n3139 = Compound Arithmetic op=MULTIPLY(0.001, w4755, w4747) -> (w4753:dbl[])
        n3140 = xnode "Read/Write Control"("FPGA VI Reference In"=w4754, "Lifetime events to read blue"=w4751) -> ("FPGA VI Reference Out"=w4757:T25)  [unwired: 1 in, 1 out]
        n3141 = call "Convert to Dynamic Data"("Array"=w4753) -> ("Dynamic Data Type"=w4752:dynamicdata)  [unwired: 3 in]
        n3142 = call "Create Histogram"("Reset"="Reset lifetime histogram", "Signal"=w4752) -> ("Histogram"=w4746:dynamicdata)  [unwired: 8 in, 1 out]
        n3143 = Equal To 0?(x=w4746) -> (x = 0?=w4745:dynamicdata)
        n3144 = xnode "Read/Write Control"("FPGA VI Reference In"=w4757, "Lifetime read blue fifo"=TRUE) -> ()  [unwired: 1 in, 2 out]
        n3145 = call "Convert from Dynamic Data"("Dynamic Data Type"=w4745) -> ("Array"=w4744:dbl[])  [unwired: 3 in]
        n3146 = Add Array Elements(numeric array=w4744) -> (sum=w4743:dbl)
        n3147 = Equal To 0?(x=w4743) -> (x = 0?=w4742:bool)
        n3148 = case shown="True" w4742 {
          tunnel: w4746 -> [w4760 w4767]
          tunnel: [w4759 w4763] -> w4740
          frame False {
            n3149 = Natural Logarithm(1:w4760) -> (0:w4759:dynamicdata)
          }
          frame True {
            n3150 = Natural Logarithm(1:w4767) -> (0:w4766:dynamicdata)
            n3151 = call "Curve Fitting"("Signals"=w4766) -> ("best fit"=w4763:dynamicdata, "slope"=w4765:dynamicdata)  [unwired: 5 in, 4 out]
            n3152 = Reciprocal(x=w4765) -> (1/x=w4764:dynamicdata)
            n3153 = Negate(x=w4764) -> (-x=w4762:dynamicdata)
            "lifetime fit (us)" <- w4762
            n3154 = call "Convert from Dynamic Data2"("Dynamic Data Type"=w4762) -> ("Array"=→"Fit lifetime vs time":dbl[])  [unwired: 3 in]
          }
        }
        n3155 = Natural Logarithm(1:w4746) -> (0:w4739:dynamicdata)
        n3156 = Merge Signals(w4739, w4740) -> (→"Fluorescence lifetime":dynamicdata)
      }
    }
    n3157 = local read "APD Elements/DMA read"() -> (w4364:u32)
    n3158 = local read "Trap AI Elements/DMA read"() -> (w4637:u32)
    n3159 = local read "Trap Pos Elements/DMA read"() -> (w4583:u32)
    n3160 = xnode "Get APD Data"("FPGA VI Reference In"=w4384, "error in"=w4584, "Number of Elements"=w4364, "Timeout (ms)"=-1) -> ("Data"=w4611:u32[], "Elements Remaining"=w4363:u32)  [unwired: 2 out]
    "APD FIFO Elements Remaining" <- w4363
    n3161 = case shown="True" "Trap positions to FIFO" {
      tunnel: w4584 -> [_ w4782]
      tunnel: w4583 -> [w4770 w4777]
      tunnel: [w4769 w4780] -> w4547
      tunnel: w4384 -> [_ w4779]
      tunnel: [FALSE w4773] -> w4357
      frame False {
        # "'Fake' data (zeros)\nNeeded when this stream is used for fluorescence lifetime measurements instead"
        n3162 = for {
          N: w4770 -> [_]
          tunnel: [u16 0] -> w4769 mode=indexing
        }
      }
      frame True {
        n3163 = xnode "Invoke Method"("FPGA VI Reference In"=w4779, "error in"=w4782, "Number of Elements"=w4777, "Timeout (ms)"=-1) -> ("Data"=w4780:u16[], "Elements Remaining"=w4776:u32)  [unwired: 2 out]
        "Trap Pos FIFO El Remaining" <- w4776
        n3164 = local read "Trap Position FIFO Depth"() -> (w4778:u32)
        n3165 = Subtract(x=w4778, y=w4777) -> (x-y=w4775:u32)
        n3166 = Divide(x=w4776, y=w4775) -> (x/y=w4772:dbl)
        "Trap positon buffer status" <- w4772
        n3167 = Equal?(x=w4772, y=1.0) -> (x = y?=w4773:bool)
      }
    }
    n3168 = local read "Number of APDs"() -> (w4453:u8)
    n3169 = xnode "Get Trap Data"("FPGA VI Reference In"=w4384, "error in"=w4584, "Number of Elements"=w4637, "Timeout (ms)"=-1 ("Timeout")) -> ("FPGA VI Reference Out"=w4482:T25, "error out"=w4481:errorcluster, "Data"=w4548:i16[], "Elements Remaining"=w4733:u32)
    "FIFO El. Rem." <- w4733
    n3170 = local read "DMA Update Period (s)"() -> (w4638:dbl)
    n3171 = local read "APD FIFO Depth"() -> (w4365:u32)
    n3172 = local read "Host fluorescence integration time (s)"() -> (w4366:dbl)
    n3173 = case "Deinterlace APD signals" shown="3, Default" w4453 {
      tunnel: [w4860 w4866] -> w4373
      tunnel: w4611 -> [w4861 w4865]
      tunnel: [w4859 w4864] -> w4371
      tunnel: [w4858 w4862] -> w4369
      frame 3, Default {
        n3174 = Decimate 1D Array "APD signals"(w4861) -> (w4860:u32[], w4859:u32[], w4858:u32[])
      }
      frame 2 {
        n3175 = Decimate 1D Array "APD signals"(w4865) -> (w4866:u32[], w4864:u32[])
        n3176 = Multiply(x=w4864, y=u32 0) -> (x*y=w4862:u32[])
      }
    }
    n3177 = local read "Trap AI FIFO Depth"() -> (w4735:u32)
    n3178 = local read "APD host processing integration"() -> (w4367:dbl)
    n3179 = Subtract(x=w4365, y=w4364) -> (x-y=w4362:u32)
    n3180 = Divide(x=w4363, y=w4362) -> (x/y=w4360:dbl)
    "APD Buffer Status" <- w4360
    n3181 = feedback #7(0.0) -> (w4576:dbl)
    n3182 = Add(x=w4638, y=w4576) -> (x+y=w4709:dbl)
    n3183 = feedback-in #7(w4709) -> ()
    n3184 = To Time Stamp(1:w4576) -> (0:w4575:timestamp)
    n3185 = Equal?(x=w4360, y=1.0) -> (x = y?=w4358:bool)
    n3186 = Subtract(x=w4735, y=w4637) -> (x-y=w4734:u32)
    n3187 = Divide(x=w4733, y=w4734) -> (x/y=w4732:dbl)
    "Buffer Status" <- w4732
    n3188 = Equal?(x=w4732, y=1.0) -> (x = y?=w4730:bool)
    n3189 = call "integrate 1D array interval - double.vi"("Ave N"=w4367, "Array In"=w4373) -> ("Array Out"=w4372:dbl[])  [unwired: 1 in]
    n3190 = call "integrate 1D array interval - double.vi"("Ave N"=w4367, "Array In"=w4371) -> ("Array Out"=w4370:dbl[])  [unwired: 1 in]
    n3191 = call "integrate 1D array interval - double.vi"("Ave N"=w4367, "Array In"=w4369) -> ("Array Out"=w4368:dbl[])  [unwired: 1 in]
    n3192 = Decimate 1D Array(w4547) -> (w4544:u16[], w4546:u16[], w4545:u16[])
    n3193 = To Unsigned Long Integer(number=w4544) -> (unsigned 32bit integer=w4543:u32[])
    n3194 = Join Numbers(hi=w4546, lo=w4545) -> ((hi.lo)=w4542:u32[])
    n3195 = Bundle("Array Out"=w4372, "Array Out"=w4370, "Array Out"=w4368) -> (w4438:T52)  [unwired: 1 in]
    n3196 = Join Numbers(hi=w4543, lo=w4542) -> ((hi.lo)=w4536:u64[])
    n3197 = Build Array(w4372, w4370, w4368) -> (w4672:dbl[][])
    n3198 = call "IR AOM word to freq - vec.vi"("Frequency Word In (double vec)"=w4536) -> ("Frequency Out"=w4582:dbl[])
    n3199 = for {
      tunnel: w4372 -> [w4856] mode=indexing
      n3200 = call "Smart Buffer (DBL) 1.vi"("new element [write]"=w4856, "mode"=T26."write") -> ()  [unwired: 4 in, 6 out]
    }
    n3201 = Decimate 1D Array(w4582) -> (w4581:dbl[], w4580:dbl[])
    n3202 = Compound Arithmetic op=OR(w4730, w4358, w4357) -> (w4361:bool)
    n3203 = case "Alert buffer overflow" shown="True" w4361 {
      frame False {
      }
      frame True {
        n3204 = call <vilib>:"Beep.vi"() -> ()  [unwired: 3 in, 9 out]
